vi "Leer escribir VIs.vi"(7 "Write? (Read)":bool, 8 "error in":errorcluster, 10 "VIs to save-Restore":string="GBL_CIU Current Program.vi", 11 "Program File Path":path=path "c:/temp.ini") -> (0 "error out":errorcluster)   [LabVIEW 2013]
uses:
  <vilib>/Utility/config.llb/NI_LVConfig.lvlib
panel:
  out "Config File Contents":string
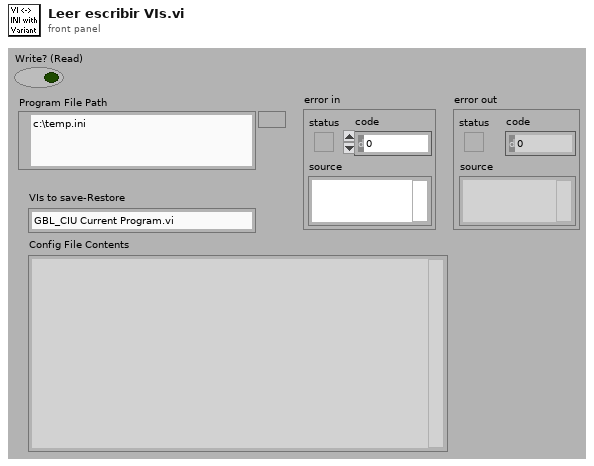
[diagram p1: front panel]
types:
  T1 = typedef "NI_LVConfig.lvlib/Config Data RefNum.ctl" = refnum<k1>
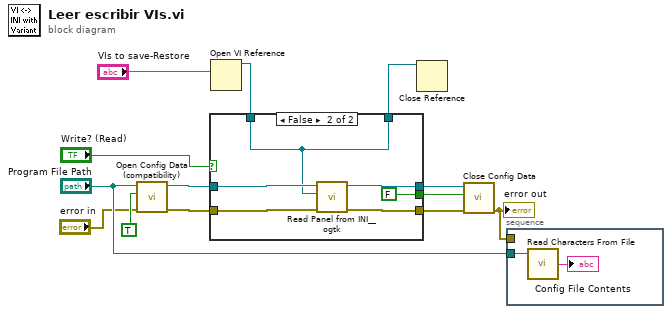
[diagram p0: block diagram]
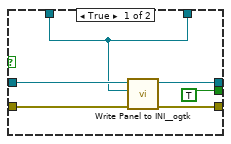
[diagram p2: hidden frame]
diagram:
  n1 = call <vilib>:"Open Config Data (compatibility).vi"("error in (no error)"="error in", "create file if necessary (T)"=TRUE ("create file if necessary? (T)"), "configuration file path"="Program File Path") -> ("error out"=w11:errorcluster, "refnum"=w13:T1)  [unwired: 6 in, 1 out]
  n2 = Open VI Reference(vi path="VIs to save-Restore") -> (vi reference=w5:refnum<vi>)  [unwired: 5 in, 1 out]
  n3 = case shown="False" "Write? (Read)" {
    tunnel: w13 -> [w19 w22]
    tunnel: [w18 w23] -> w12
    tunnel: w11 -> [w17 w25]
    tunnel: [w16 w24] -> w10
    tunnel: w5 -> [w15 w21]
    tunnel: [w15 w21] -> w4
    tunnel: [TRUE ("write configuration file? (F)") FALSE ("write configuration file? (F)")] -> w3
    frame True {
      n4 = call "Write Panel to INI__ogtk.vi"("error in (no error)"=w17, "VI ref"=w15, "refnum"=w19) -> ("error out"=w16:errorcluster, "refnum out"=w18:T1)  [unwired: 7 in]
    }
    frame False {
      n5 = call "Read Panel from INI__ogtk.vi"("error in (no error)"=w25, "VI ref"=w21, "refnum"=w22) -> ("error out"=w24:errorcluster, "refnum out"=w23:T1)  [unwired: 7 in]
    }
  }
  n6 = Close Reference(reference=w4) -> ()  [unwired: 1 in, 1 out]
  n7 = call <vilib>:"Close Config Data.vi"("error in (no error)"=w10, "write file if changed (T)"=w3, "refnum"=w12) -> ("error out"=w6:errorcluster)  [unwired: 7 in, 1 out]
  "error out" <- w6
  n8 = stacked-sequence {
    tunnel: "Program File Path" -> [w26]
    tunnel: w6 -> [_]
    frame #0 {
      n9 = call <vilib>:"Read Characters From File.vi"("file path (dialog if empty)"=w26) -> ("character string"=→"Config File Contents":string)  [unwired: 5 in, 3 out]
    }
  }
